vi "TablerRole.vi"(6 "Tactic index in":i32, 7 "first call":bool, 8 "error in (no error)":errorcluster, 10 "Game in":refnum<class "Game.lvclass">, 11 "TablerRole in":refnum<class "TablerRole.lvclass">) -> (0 "error out":errorcluster, 1 "tactic index":i32, 2 "Robot out":refnum<class "Robot.lvclass">, 3 "TablerRole out":refnum<class "TablerRole.lvclass">)   [LabVIEW 2018, in "TablerRole.lvclass"]
uses:
  TablerRole.lvclass
  Game_class/Game.lvclass
  Robot_class/Robot.lvclass
  Role_class/Role.lvclass/Role.ctl
  TablerRole.lvclass/TablerRole.ctl
  Tacticbook_class/Tacticbook.lvclass/Tacticbook.ctl
  FollowAttackerTactic_class/FollowAttackerTactic.lvclass/FollowAttackerTactic.ctl
  Tacticbook_class/Read WaitPassTactic.vi
  Tacticbook_class/Write WaitPassTactic.vi
  Tacticbook_class/Read FollowAttackerTactic.vi
  FollowAttackerTactic_class/Read States.vi
  Tacticbook_class/Write FollowAttackerTactic.vi
  Role_class/Read Tacticbook.vi
  Read number_of_tactics.vi
  Role_class/Write Tacticbook.vi
  Role_class/Write tactic_index.vi
  Role_class/Read RobotRef.vi
  Tacticbook_class/Tacticbook.lvclass
  WaitPassTactic_class/WaitPassTactic.lvclass
  KickToPassReceiverTactic_class/KickToPassReceiverTactic.lvclass
  FollowAttackerTactic_class/FollowAttackerTactic.lvclass
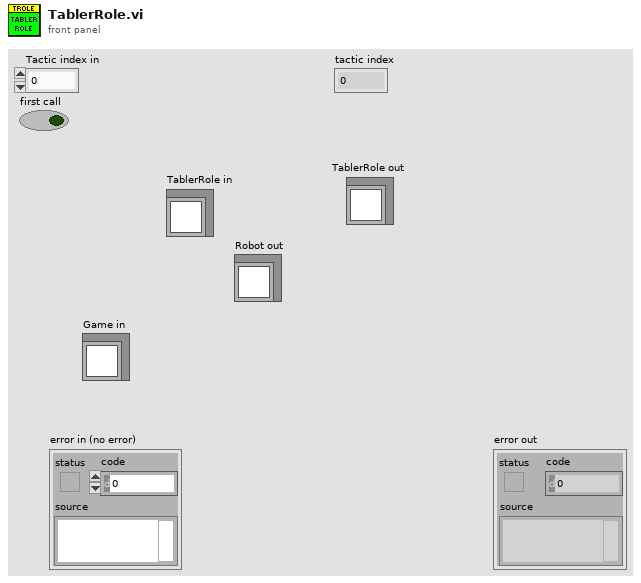
[diagram p1: front panel]
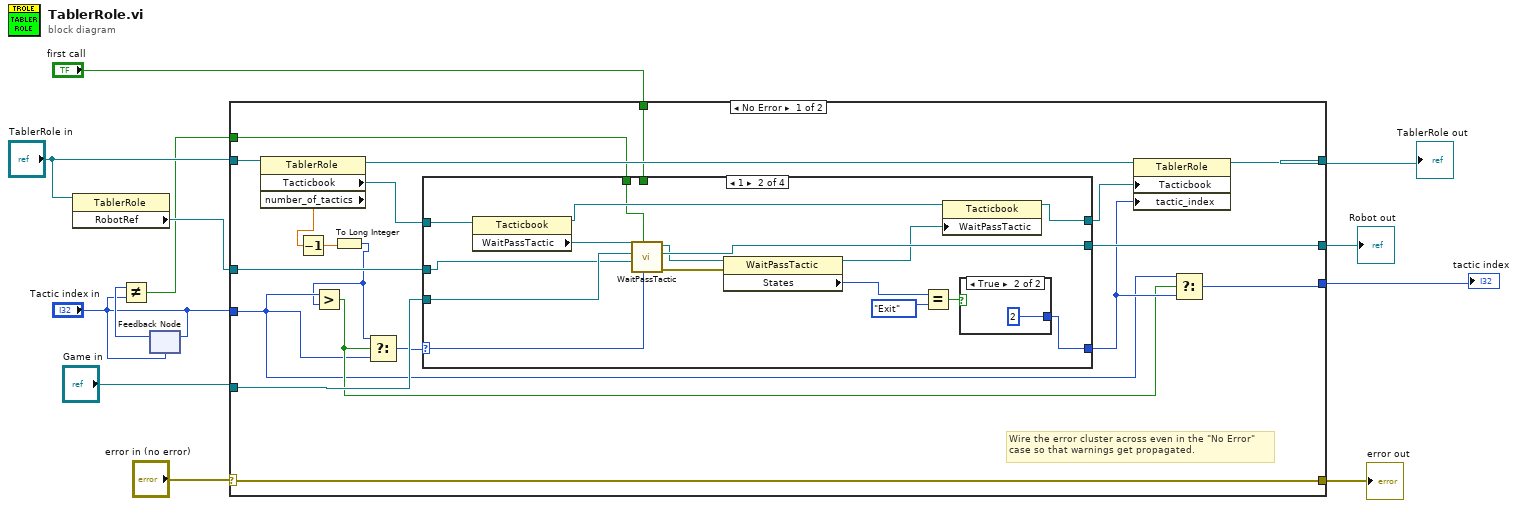
[diagram p0: block diagram]
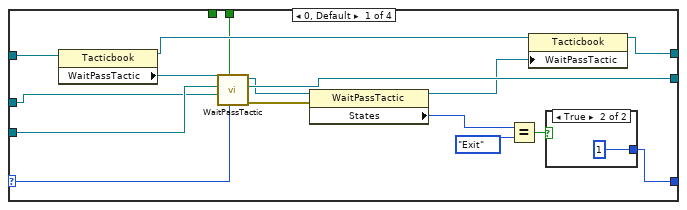
[diagram p2: hidden frame]
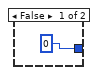
[diagram p3: hidden frame]
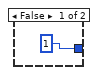
[diagram p4: hidden frame]
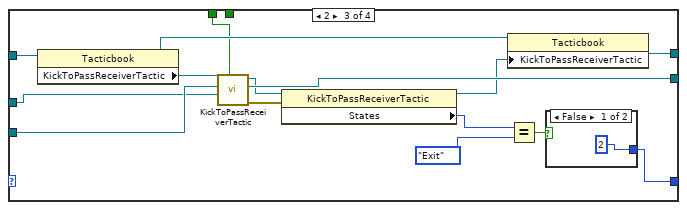
[diagram p5: hidden frame]
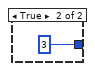
[diagram p6: hidden frame]
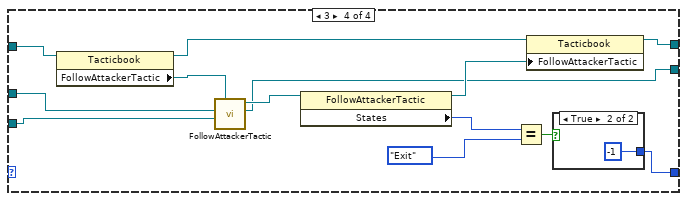
[diagram p7: hidden frame]
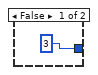
[diagram p8: hidden frame]
diagram:
  n1 = property class="TablerRole"(reference="TablerRole in") -> ("RobotRef"=w10:refnum<class "Robot.lvclass">)  [unwired: 1 in, 2 out]
  n2 = feedback-in #1("Tactic index in") -> ()
  n3 = feedback #1("Tactic index in") -> (w4:i32)
  n4 = Not Equal?(x=w4, y="Tactic index in") -> (x != y?=w2:bool)
  n5 = case shown="No Error" "error in (no error)" {
    selector: "error in (no error)" -> [w31 w102]
    tunnel: [w31 w102] -> w11
    tunnel: [w29 w101] -> w8
    tunnel: "TablerRole in" -> [w30 w101]
    tunnel: w10 -> [w26 w100]
    tunnel: [w25 w100] -> w1
    tunnel: "Game in" -> [w23 _]
    tunnel: [w21 _] -> w7
    tunnel: "Tactic index in" -> [w18 _]
    tunnel: "first call" -> [w16 _]
    tunnel: w2 -> [w13 _]
    frame No Error {
      # "Wire the error cluster across even in the \"No Error\"\ncase so that warnings get propagated."
      n6 = property class="TablerRole"(reference=w30) -> (reference out=w28:refnum<class "TablerRole.lvclass">, "Tacticbook"=w27:refnum<class "Tacticbook.lvclass">, "number_of_tactics"=w17:dbl)  [unwired: 1 in, 1 out]
      n7 = Decrement(x=w17) -> (x-1=w15:dbl)
      n8 = To Long Integer(number=w15) -> (32bit integer=w14:i32)
      n9 = Greater?(x=w18, y=w14) -> (0:w19:bool)
      n10 = Select(t=w14, s=w19, f=w18) -> (s? t:f=w20:i32)
      n11 = case shown="1" w20 {
        selector: w20 -> [w32 w50 _ _]
        tunnel: [w35 w53 w70 w86] -> w22
        tunnel: w27 -> [w47 w65 w82 w95]
        tunnel: w26 -> [w38 w56 w73 w88]
        tunnel: [w46 w64 w81 w89] -> w25
        tunnel: [w42 w60 w77 w93] -> w24
        tunnel: w23 -> [w39 w57 w74 w87]
        tunnel: w16 -> [w34 _ _ _]
        tunnel: w13 -> [_ w52 w68 _]
        frame 0, Default {
          n12 = property class="Tacticbook"(reference=w47) -> (reference out=w44:refnum<class "Tacticbook.lvclass">, "WaitPassTactic"=w41:refnum<class "WaitPassTactic.lvclass">)  [unwired: 1 in, 1 out]
          n13 = call-dynamic "WaitPassTactic.vi"("Tactic index in"=w32, "first call"=w34, "Robot"=w38, "Game in"=w39, "WaitPassTactic in"=w41) -> ("error out"=w45:errorcluster, "Robot out"=w46:refnum<class "Robot.lvclass">, "WaitPassTactic out"=w40:refnum<class "WaitPassTactic.lvclass">)  [unwired: 4 in]
          n14 = property class="WaitPassTactic"(reference=w40, error in=w45) -> (reference out=w43:refnum<class "WaitPassTactic.lvclass">, "States"=w36:enum16{"State 0", "State 1", "State 2", "Exit"})  [unwired: 1 out]
          n15 = Equal?(x=w36, y=enum16{"State 0", "State 1", "State 2", "Exit"}."Exit") -> (x = y?=w37:bool)
          n16 = property class="Tacticbook"(reference=w44, "WaitPassTactic"=w43) -> (reference out=w42:refnum<class "Tacticbook.lvclass">)  [unwired: 1 in, 1 out]
          n17 = case shown="True" w37 {
            tunnel: [0 1] -> w35
            frame False {
            }
            frame True {
            }
          }
        }
        frame 1 {
          n18 = property class="Tacticbook"(reference=w65) -> (reference out=w62:refnum<class "Tacticbook.lvclass">, "WaitPassTactic"=w59:refnum<class "WaitPassTactic.lvclass">)  [unwired: 1 in, 1 out]
          n19 = call-dynamic "WaitPassTactic.vi"("Tactic index in"=w50, "first call"=w52, "Robot"=w56, "Game in"=w57, "WaitPassTactic in"=w59) -> ("error out"=w63:errorcluster, "Robot out"=w64:refnum<class "Robot.lvclass">, "WaitPassTactic out"=w58:refnum<class "WaitPassTactic.lvclass">)  [unwired: 4 in]
          n20 = property class="WaitPassTactic"(reference=w58, error in=w63) -> (reference out=w61:refnum<class "WaitPassTactic.lvclass">, "States"=w54:enum16{"State 0", "State 1", "State 2", "Exit"})  [unwired: 1 out]
          n21 = Equal?(x=w54, y=enum16{"State 0", "State 1", "State 2", "Exit"}."Exit") -> (x = y?=w55:bool)
          n22 = property class="Tacticbook"(reference=w62, "WaitPassTactic"=w61) -> (reference out=w60:refnum<class "Tacticbook.lvclass">)  [unwired: 1 in, 1 out]
          n23 = case shown="True" w55 {
            tunnel: [1 2] -> w53
            frame False {
            }
            frame True {
            }
          }
        }
        frame 2 {
          n24 = property class="Tacticbook"(reference=w82) -> (reference out=w79:refnum<class "Tacticbook.lvclass">, "KickToPassReceiverTactic"=w76:refnum<class "KickToPassReceiverTactic.lvclass">)  [unwired: 1 in, 1 out]
          n25 = call "KickToPassReceiverTactic.vi"("first call"=w68, "Robot"=w73, "Game in"=w74, "KickToPassReceiverTactic in"=w76) -> ("error out"=w80:errorcluster, "Robot out"=w81:refnum<class "Robot.lvclass">, "KickToPassReceiverTactic out"=w75:refnum<class "KickToPassReceiverTactic.lvclass">)  [unwired: 5 in]
          n26 = property class="KickToPassReceiverTactic"(reference=w75, error in=w80) -> (reference out=w78:refnum<class "KickToPassReceiverTactic.lvclass">, "States"=w71:enum16{"KickToPassReceiver", "WaitPass", "Exit"})  [unwired: 1 out]
          n27 = property class="Tacticbook"(reference=w79, "KickToPassReceiverTactic"=w78) -> (reference out=w77:refnum<class "Tacticbook.lvclass">)  [unwired: 1 in, 1 out]
          n28 = Equal?(x=w71, y=enum16{"KickToPassReceiver", "WaitPass", "Exit"}."Exit") -> (x = y?=w72:bool)
          n29 = case shown="False" w72 {
            tunnel: [2 3] -> w70
            frame False {
            }
            frame True {
            }
          }
        }
        frame 3 {
          n30 = property class="Tacticbook"(reference=w95) -> (reference out=w94:refnum<class "Tacticbook.lvclass">, "FollowAttackerTactic"=w91:refnum<class "FollowAttackerTactic.lvclass">)  [unwired: 1 in, 1 out]
          n31 = call-dynamic "FollowAttackerTactic.vi"("Game in"=w87, "Robot"=w88, "FollowAttackerTactic in"=w91) -> ("Robot out"=w89:refnum<class "Robot.lvclass">, "FollowAttackerTactic out"=w90:refnum<class "FollowAttackerTactic.lvclass">)  [unwired: 6 in, 1 out]
          n32 = property class="FollowAttackerTactic"(reference=w90) -> (reference out=w92:refnum<class "FollowAttackerTactic.lvclass">, "States"=w96:enum16{"Exit", "FollowAttacker"})  [unwired: 1 in, 1 out]
          n33 = Equal?(x=w96, y=enum16{"Exit", "FollowAttacker"}."Exit" ("States")) -> (x = y?=w97:bool)
          n34 = property class="Tacticbook"(reference=w94, "FollowAttackerTactic"=w92) -> (reference out=w93:refnum<class "Tacticbook.lvclass">)  [unwired: 1 in, 1 out]
          n35 = case shown="True" w97 {
            tunnel: [3 -1] -> w86
            frame False {
            }
            frame True {
            }
          }
        }
      }
      n36 = property class="TablerRole"(reference=w28, "Tacticbook"=w24, "tactic_index"=w22) -> (reference out=w29:refnum<class "TablerRole.lvclass">)  [unwired: 1 in, 1 out]
      n37 = Select(t=w18, s=w19, f=w22) -> (s? t:f=w21:i32)
    }
    frame Error {
    }
  }
  "error out" <- w11
  "TablerRole out" <- w8
  "tactic index" <- w7
  "Robot out" <- w1
